vi "peak_value_calculate_A_4_v1.vi"(0 "IO Module\\AI 1 Data N-1 2":i16, 1 "IO Module\\AI 1 Data N-2 3":i16, 2 "IO Module\\AI 1 Data N-2 2":i16, 3 "Boolean in":bool, 4 "IO Module\\AI 1 Data N-3 2":i16, 6 "IO Module\\AI 1 Data N 3":i16, 7 "IO Module\\AI 1 Data N":i16, 8 "IO Module\\AI 1 Data N-1 3":i16, 9 "IO Module\\AI 1 Data N-3":i16, 10 "IO Module\\AI 1 Data N 2":i16, 11 "IO Module\\AI 1 Data N-1":i16, 13 "IO Module\\AI 1 Data N-2":i16) -> (15 "Read Ready":bool, 16 "Spike Value":i16)   [LabVIEW 2020]
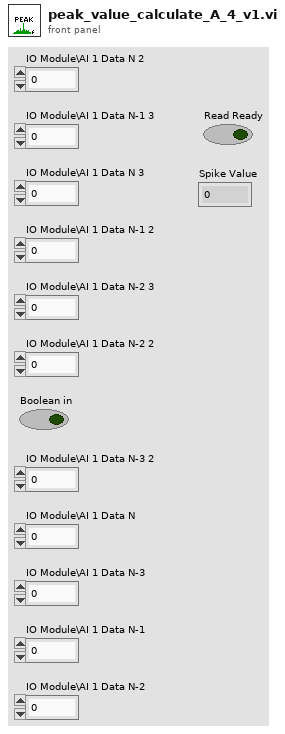
[diagram p1: front panel]
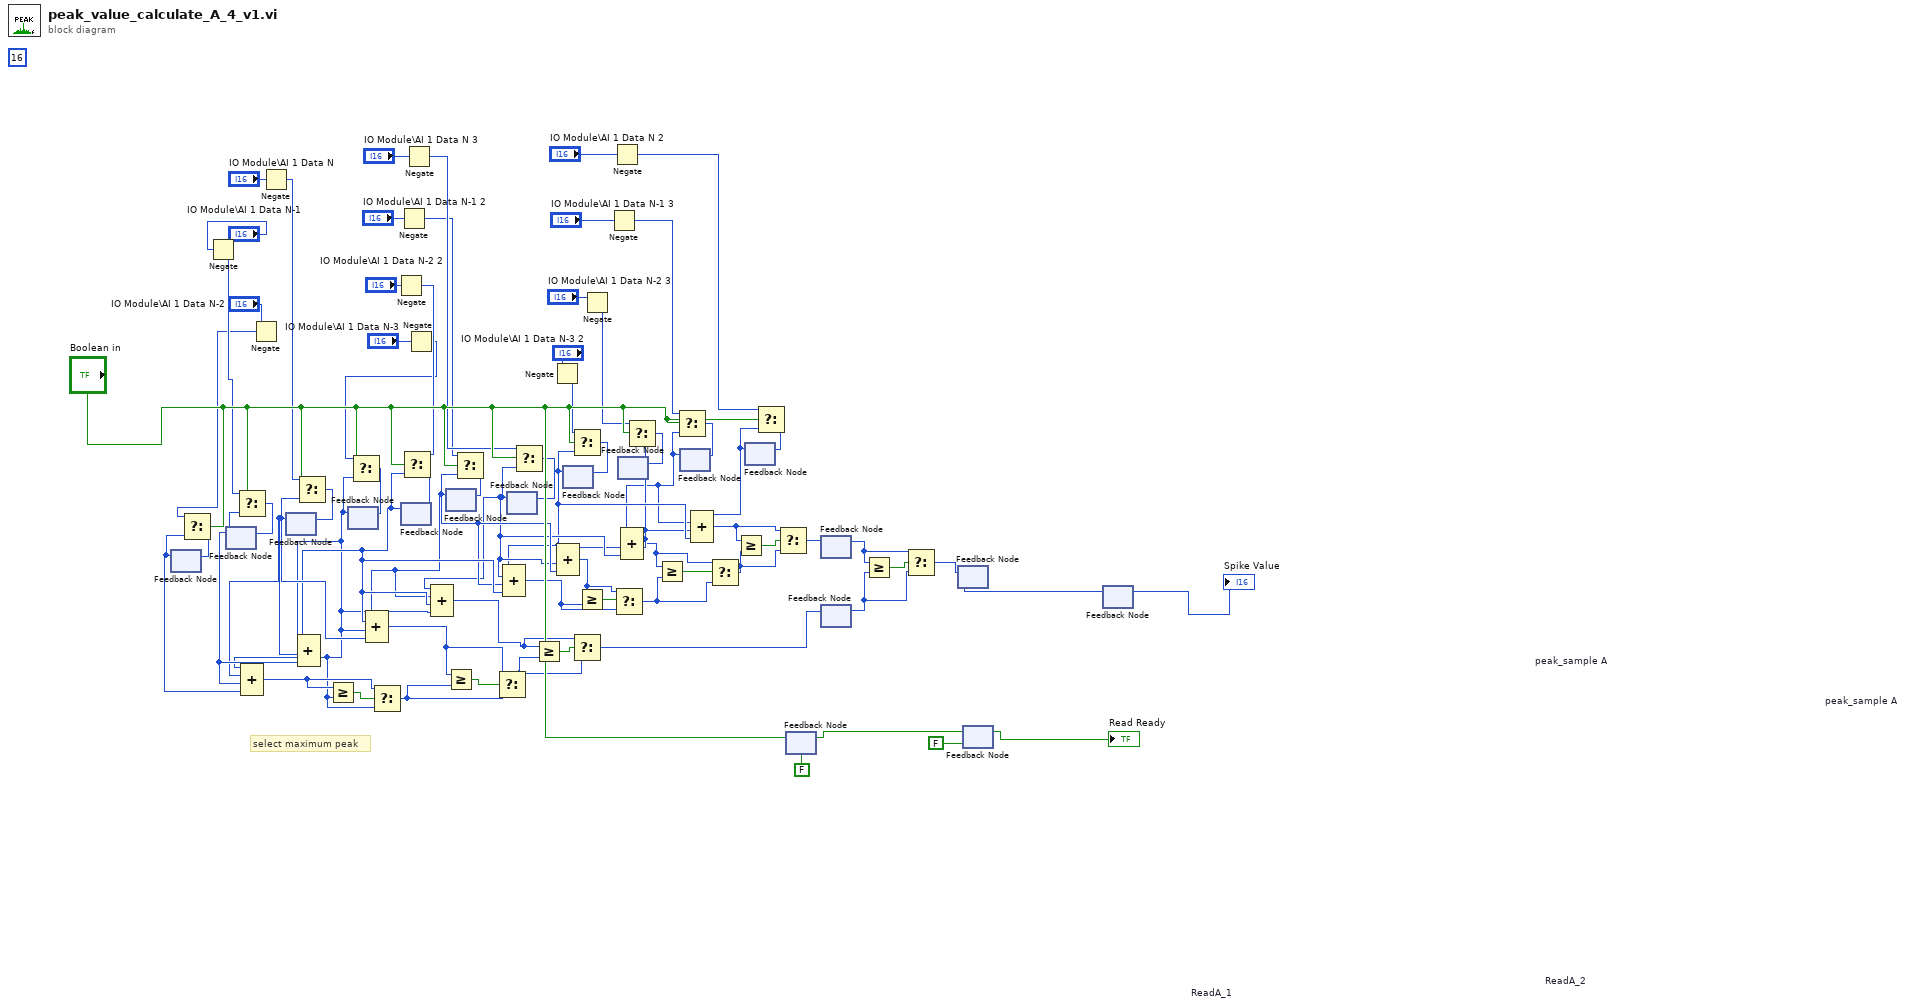
[diagram p0: block diagram]
diagram:
  (unwired) 16
  # "select maximum peak"
  n1 = feedback #1() -> (w44:i16)  [unwired: 1 in]
  n2 = Negate(x="IO Module\\AI 1 Data N-1") -> (-x=w31:i16)
  n3 = feedback #2() -> (w43:i16)  [unwired: 1 in]
  n4 = Select(t=w31, s="Boolean in", f=w43) -> (s? t:f=w54:i16)
  n5 = feedback-in #2(w54) -> ()
  n6 = Negate(x="IO Module\\AI 1 Data N-2") -> (-x=w30:i16)
  n7 = Select(t=w30, s="Boolean in", f=w44) -> (s? t:f=w65:i16)
  n8 = feedback-in #1(w65) -> ()
  n9 = Negate(x="IO Module\\AI 1 Data N") -> (-x=w32:i16)
  n10 = feedback #3() -> (w29:i16)  [unwired: 1 in]
  n11 = Select(t=w32, s="Boolean in", f=w29) -> (s? t:f=w55:i16)
  n12 = feedback-in #3(w55) -> ()
  n13 = feedback #4() -> (w19:i16)  [unwired: 1 in]
  n14 = Compound Arithmetic op=ADD(w19, w29, w43, w44) -> (w20:i16)
  n15 = Greater Or Equal?(x=w20, y=w19) -> (x >= y?=w21:bool)
  n16 = Select(t=w20, s=w21, f=w19) -> (s? t:f=w67:i16)
  n17 = Negate(x="IO Module\\AI 1 Data N-2 2") -> (-x=w34:i16)
  n18 = Negate(x="IO Module\\AI 1 Data N-1 2") -> (-x=w35:i16)
  n19 = feedback #5() -> (w28:i16)  [unwired: 1 in]
  n20 = Compound Arithmetic op=ADD(w28, w19, w29, w43) -> ()  [unwired: 1 out]
  n21 = Select(t=w34, s="Boolean in", f=w28) -> (s? t:f=w61:i16)
  n22 = feedback-in #5(w61) -> ()
  n23 = Negate(x="IO Module\\AI 1 Data N 3") -> (-x=w36:i16)
  n24 = Negate(x="IO Module\\AI 1 Data N-3") -> (-x=w33:i16)
  n25 = Select(t=w33, s="Boolean in", f=w19) -> (s? t:f=w66:i16)
  n26 = feedback-in #4(w66) -> ()
  n27 = feedback #6() -> (w27:i16)  [unwired: 1 in]
  n28 = Compound Arithmetic op=ADD(w27, w28, w19, w29) -> (w18:i16)
  n29 = Greater Or Equal?(x=w18, y=w67) -> (x >= y?=w68:bool)
  n30 = Select(t=w35, s="Boolean in", f=w27) -> (s? t:f=w62:i16)
  n31 = feedback-in #6(w62) -> ()
  n32 = Select(t=w18, s=w68, f=w67) -> (s? t:f=w15:i16)
  n33 = feedback #7() -> (w26:i16)  [unwired: 1 in]
  n34 = Compound Arithmetic op=ADD(w26, w27, w28, w19) -> (w16:i16)
  n35 = Select(t=w36, s="Boolean in", f=w26) -> (s? t:f=w63:i16)
  n36 = feedback-in #7(w63) -> ()
  n37 = Greater Or Equal?(x=w16, y=w15) -> (x >= y?=w17:bool)
  n38 = Negate(x="IO Module\\AI 1 Data N-3 2") -> (-x=w37:i16)
  n39 = feedback #8() -> (w25:i16)  [unwired: 1 in]
  n40 = Compound Arithmetic op=ADD(w25, w26, w27, w28) -> (w13:i16)
  n41 = Select(t=w37, s="Boolean in", f=w25) -> (s? t:f=w49:i16)
  n42 = feedback-in #8(w49) -> ()
  n43 = Select(t=w16, s=w17, f=w15) -> (s? t:f=w14:i16)
  n44 = Negate(x="IO Module\\AI 1 Data N-2 3") -> (-x=w38:i16)
  n45 = Negate(x="IO Module\\AI 1 Data N-1 3") -> (-x=w39:i16)
  n46 = Negate(x="IO Module\\AI 1 Data N 2") -> (-x=w40:i16)
  n47 = feedback #9() -> (w24:i16)  [unwired: 1 in]
  n48 = Compound Arithmetic op=ADD(w24, w25, w26, w27) -> (w12:i16)
  n49 = Greater Or Equal?(x=w12, y=w13) -> (x >= y?=w69:bool)
  n50 = Select(t=w12, s=w69, f=w13) -> (s? t:f=w70:i16)
  n51 = Select(t=w38, s="Boolean in", f=w24) -> (s? t:f=w47:i16)
  n52 = feedback-in #9(w47) -> ()
  n53 = feedback #10() -> (w23:i16)  [unwired: 1 in]
  n54 = Compound Arithmetic op=ADD(w23, w24, w24, w26) -> (w11:i16)
  n55 = Greater Or Equal?(x=w11, y=w70) -> (x >= y?=w71:bool)
  n56 = Select(t=w39, s="Boolean in", f=w23) -> (s? t:f=w45:i16)
  n57 = feedback-in #10(w45) -> ()
  n58 = Select(t=w11, s=w71, f=w70) -> (s? t:f=w8:i16)
  n59 = feedback #11() -> (w22:i16)  [unwired: 1 in]
  n60 = Compound Arithmetic op=ADD(w22, w23, w24, w25) -> (w9:i16)
  n61 = Greater Or Equal?(x=w9, y=w8) -> (x >= y?=w10:bool)
  n62 = Select(t=w40, s="Boolean in", f=w22) -> (s? t:f=w57:i16)
  n63 = feedback-in #11(w57) -> ()
  n64 = Select(t=w9, s=w10, f=w8) -> (s? t:f=w7:i16)
  n65 = feedback #12 "ReadA_1"(FALSE ("Boolean in")) -> (w73:bool)
  n66 = feedback-in #12("Boolean in") -> ()
  n67 = feedback #13() -> (w5:i16)  [unwired: 1 in]
  n68 = feedback-in #13(w7) -> ()
  n69 = feedback #14() -> (w4:i16)  [unwired: 1 in]
  n70 = feedback-in #14(w14) -> ()
  n71 = Greater Or Equal?(x=w5, y=w4) -> (x >= y?=w6:bool)
  n72 = Select(t=w5, s=w6, f=w4) -> (s? t:f=w3:i16)
  n73 = feedback #15 "peak_sample A"() -> (w74:i16)  [unwired: 1 in]
  n74 = feedback-in #15(w3) -> ()
  n75 = feedback #16 "ReadA_2"(FALSE ("Boolean in")) -> (→"Read Ready":bool)
  n76 = feedback-in #16(w73) -> ()
  n77 = feedback #17 "peak_sample A"() -> (→"Spike Value":i16)  [unwired: 1 in]
  n78 = feedback-in #17(w74) -> ()
